vi "Feed.vi"() -> ()   [LabVIEW 2013]
panel:
  out "Long Average":dbl
  out "Fine Avg":dbl
  out "FQ":cluster{dbl, dbl}(graph)
  out "Front Pannel":dbl[](graph)
  out "FeedRate":dbl
  in  "Feeder Op":bool
  out "Balance":dbl
  in  "Auto Voltage":bool
  in  "XV-202":bool
  out "Feed DP":dbl format="%.1f"
  out "V-200 O2":dbl format="%.1f"
  out "Feed Hopper":dbl(slide) scale=75.0..100.0
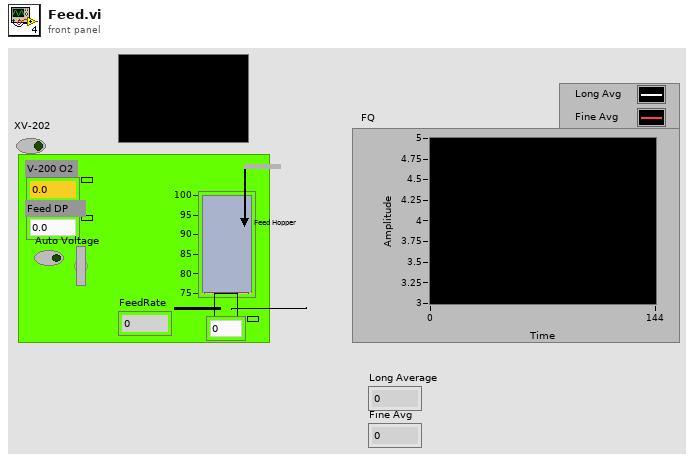
[diagram p1: front panel]
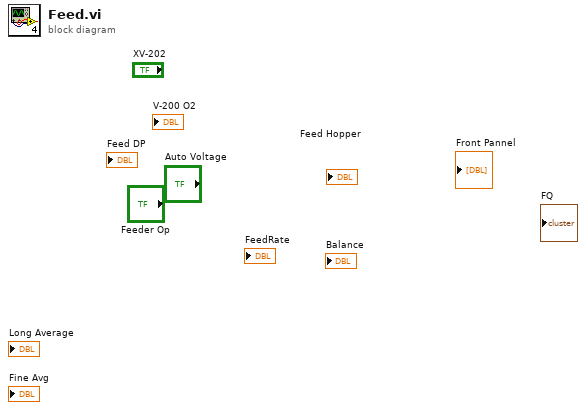
[diagram p0: block diagram]
diagram:
